vi "Globals.vi"() -> ()   [LabVIEW 2014]
uses:
  STD - Tap Mode.ctl
  <vilib>/LabVIEW Hacker/LINX/Private/Type Defs/LINX Ref.ctl
  <vilib>/LabVIEW Hacker/LINX/Private/Type Defs/Platform.ctl
  <vilib>/LabVIEW Hacker/LINX/Private/Type Defs/Interface.ctl
  <vilib>/LabVIEW Hacker/LINX/Private/Device/Type Defs/LINX Device Config.ctl
  <vilib>/LabVIEW Hacker/LINX/Private/Device/Type Defs/TCP Config.ctl
  <vilib>/LabVIEW Hacker/LINX/Private/Type Defs/Device Family.ctl
  <vilib>/userdefined/High Color/IMAQdx.ctl
  ImageCluster.ctl
  <vilib>/vision/Image Controls.llb/IMAQ Image.ctl
  FlappyHeightPoint.ctl
  <vilib>/LabVIEW Hacker/LINX/LVH-LINX.lvlib
  <vilib>/LabVIEW Hacker/LINX/Private/Device/Device.lvlib
panel:
  in  "Tab Control":T1(tab)
  in  "Tap pin":u32
  in  "Horizontal scroll speed (px/s)":dbl
  in  "Pipe width":u32
  in  "Flappy acceleration":dbl
  in  "Post-tap velocity":dbl
  in  "Stay-level time":dbl
  in  "Flappy left offset":u32
  in  "Start time offset":dbl
  in  "Last tap time":dbl
  in  "Image height":u32
  in  "Image width":u32
  in  "FlappyHeightHistory":T2[](array[typedef])
  in  "LINX Resource":T3
  in  "IMAQdx Camera Session":T9
  in  "Flappy Template":T10
  in  "Pipe Template":T10
  in  "Display Screen":T10
  in  "Image Queue":refnum<queue>
  in  "Error Queue":refnum<queue>
  out "Play":bool
  out "Image aligned?":bool
  out "all stop":bool
  in  "Control Mode":T11
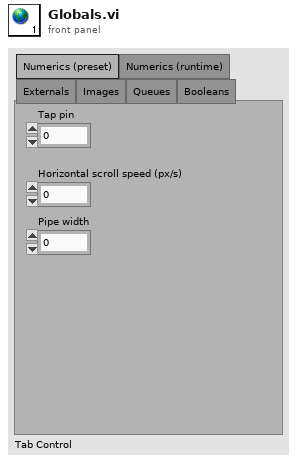
[diagram p1: front panel]
types:
  T1 = enum32{"Numerics (preset)", "Numerics (runtime)", "Externals", "Images", "Queues", "Booleans"}
  T2 = typedef "FlappyHeightPoint.ctl" = cluster{"Time (s)":dbl, "Height (px)":dbl}
  T3 = typedef "LVH-LINX.lvlib/LINX Ref.ctl" = cluster{"Platform":T4, "Interface":T5, "LINX Device Config":T6}
  T4 = typedef "LVH-LINX.lvlib/Platform.ctl" = enum16{"LINX", "myRIO"}
  T5 = typedef "LVH-LINX.lvlib/Interface.ctl" = enum16{"Serial", "TCP"}
  T6 = typedef "LVH-LINX.lvlib/Device.lvlib/LINX Device Config.ctl" = cluster{"Interface":T5, "COM Port":refnum<visa-resource-name>, "TCP Configuration":T7, "Device Family":T8, "Device ID":u8, "Device Name":string, "TCP Ref":refnum<k5>}
  T7 = typedef "LVH-LINX.lvlib/Device.lvlib/TCP Config.ctl" = cluster{"IP Address":string, "Port":u16}
  T8 = typedef "LVH-LINX.lvlib/Device Family.ctl" = enum8{"National Instruments", "Digilent", "Arduino"}
  T9 = typedef "IMAQdx.ctl" = refnum<k21>
  T10 = typedef "IMAQ Image.ctl" = refnum<image>
  T11 = typedef "STD - Tap Mode.ctl" = enum32{"No Action", "Stay Level", "Rise", "Fall", "Calibrate"}
diagram:
